vi "Create user Defind Error code.vi"(10 "error in (no Error)":errorcluster, 11 "User Defind Code":i32) -> (2 "Error Output":errorcluster)   [LabVIEW 2021]
doc: "创建错误，仅仅输入自定义的错误代码。具体含义，在Error模块里面通过读取csv文件得到。\n2014-09-24 15:31:26\n蒋松\njiangsong@outlook.com"
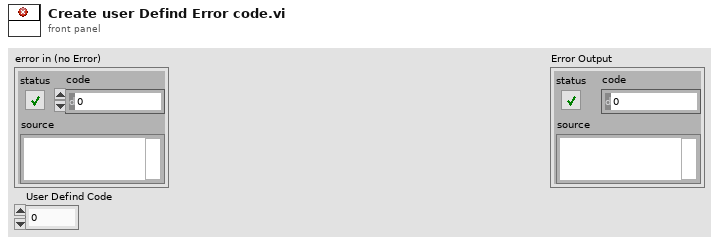
[diagram p1: front panel]
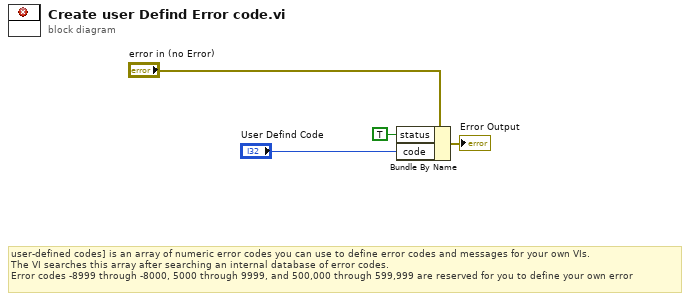
[diagram p0: block diagram]
diagram:
  # "user-defined codes] is an array of numeric error codes you can use to define error codes and messages for your own VIs. \nThe VI searches this array after searching an internal database of error codes. \nError codes -8999 through -8000, 5000 through 9999, and 500,000 through 599,999 are reserved for you to define your own error"
  n1 = Bundle By Name(cluster="error in (no Error)", "status"=TRUE, "code"="User Defind Code") -> (→"Error Output":errorcluster)
